vi "Next.vi"(7 "Previous In":refnum<class "Known Host.lvclass">, 8 "Error In":errorcluster, 10 "Next In":refnum<class "Known Host.lvclass">, 11 "Known Hosts In":refnum<class "Known Hosts.lvclass">) -> (0 "Error Out":errorcluster, 1 "Result":T1 items=["Success", "End of Hosts"], 2 "Next Out":refnum<class "Known Host.lvclass">, 3 "Known Hosts Out":refnum<class "Known Hosts.lvclass">, 5 "Previous Out":refnum<class "Known Host.lvclass">)   [LabVIEW 2018, in "Toolkit.lvlib" / "Known Hosts.lvclass"]
doc: "Gets the next known host in an internal libssh2lv shared library linked list represented by this Known Hosts object."
uses:
  Known Hosts.lvclass
  Known Host/Known Host.lvclass
  Type Definitions/Get Results.ctl
  Known Hosts.lvclass/Known Hosts.ctl
  Known Host/Known Host.lvclass/Known Host.ctl
  Session/Session.lvclass/Session.ctl
  SSH/SSH.lvclass/SSH.ctl
  Toolkit.lvlib
  Session/Session.lvclass
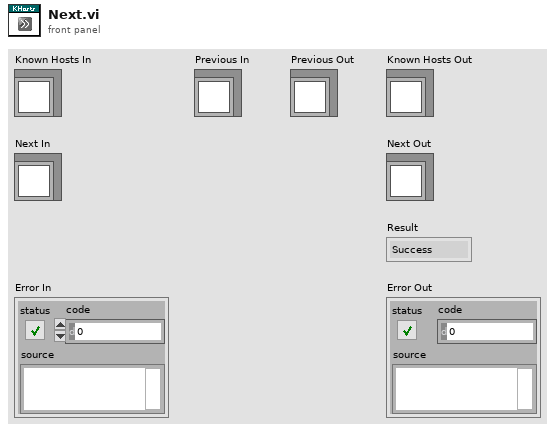
[diagram p1: front panel]
types:
  T1 = typedef "Toolkit.lvlib/Known Hosts.lvclass/Get Results.ctl" = i32
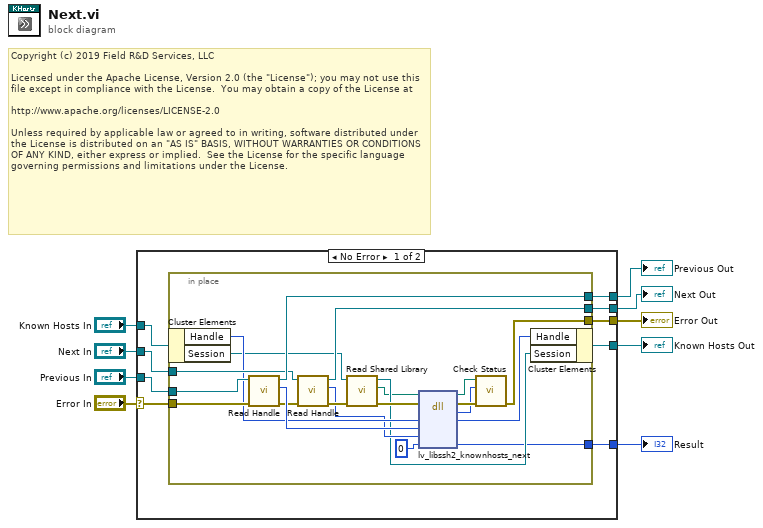
[diagram p0: block diagram]
diagram:
  # "Copyright (c) 2019 Field R&D Services, LLC\n\nLicensed under the Apache License, Version 2.0 (the \"License\"); you may not use this file except in compliance with the License.  You may obtain a copy of the License at\n\nhttp://www.apache.org/licenses/LICENSE-2.0\n\nUnless required by applicable law or agreed to in writing, software distributed under the License is distributed on an \"AS IS\" BASIS, WITHOUT WARRANTIES OR CONDITIONS OF ANY KIND, either express or implied.  See the License for the specific language governing permissions and limitations under the License."
  n1 = case shown="No Error" "Error In" {
    selector: "Error In" -> [w17 w43]
    tunnel: "Known Hosts In" -> [w18 w42]
    tunnel: [w16 w43] -> w7
    tunnel: [w11 w42] -> w6
    tunnel: "Previous In" -> [w15 w41]
    tunnel: [w14 w41] -> w4
    tunnel: "Next In" -> [w13 w40]
    tunnel: [w12 w40] -> w2
    tunnel: [w10 _] -> w1
    frame No Error {
      n2 = in-place {
        in-place-border: w17 -> [w33]
        in-place-border: [w36] -> w16
        in-place-border: w15 -> [w34]
        in-place-border: [w31] -> w14
        in-place-border: w13 -> [w28]
        in-place-border: [w27] -> w12
        in-place-border: [w19] -> w10
        n3 = in-place-cluster #1(w18) -> ("Handle"=w26:u64, "Session"=w22:refnum<class "Session.lvclass">)
        n4 = call "Read Handle.vi"("Error In"=w33, "Known Host In"=w34) -> ("Error Out"=w29:errorcluster, "Handle"=w32:u64, "Known Host Out"=w31:refnum<class "Known Host.lvclass">)  [unwired: 7 in]
        n5 = call "Read Handle.vi"("Error In"=w29, "Known Host In"=w28) -> ("Error Out"=w25:errorcluster, "Handle"=w24:u64, "Known Host Out"=w27:refnum<class "Known Host.lvclass">)  [unwired: 7 in]
        n6 = call "Read Shared Library.vi"("Error In"=w25, "Session In"=w22) -> ("Erorr Out"=w23:errorcluster, "libssh2lv Shared Library"=w20:path, "Session Out"=w21:refnum<class "Session.lvclass">)  [unwired: 7 in]
        n7 = dll-call lib="lv-libssh2.*" fn="lv_libssh2_knownhosts_next"(path in=w20, error in=w23, "handle"=w26, "previous"=w32, "next"=w24, "result"=0) -> (path out=w37:path, error out=w38:errorcluster, "status"=w35:i32, "handle"=w39:u64, "result"=w19:i32)  [unwired: 3 in]
        n8 = call "Check Status.vi"("Error In"=w38, "Status"=w35, "libssh2lv Shared Library In"=w37) -> ("Error Out"=w36:errorcluster)  [unwired: 7 in, 1 out]
        n9 = in-place-cluster #1("Handle"=w39, "Session"=w21) -> (w11:refnum<class "Known Hosts.lvclass">)
      }
    }
    frame Error {
    }
  }
  "Error Out" <- w7
  "Known Hosts Out" <- w6
  "Previous Out" <- w4
  "Result" <- w1
  "Next Out" <- w2
